vi "Writetofile.vi"(3 "error in (no error)":errorcluster, 4 "Componenet":string, 5 "Write":bool, 6 "Card":i32) -> (0 "error out":errorcluster)   [LabVIEW 2011]
doc: "The vi are saving the current circuit configuration.\n\nThe port White are enable/disable writing to the file, False --> disable writing, True --> enable writing.\n\nThe file are saved on Current VI's Path."
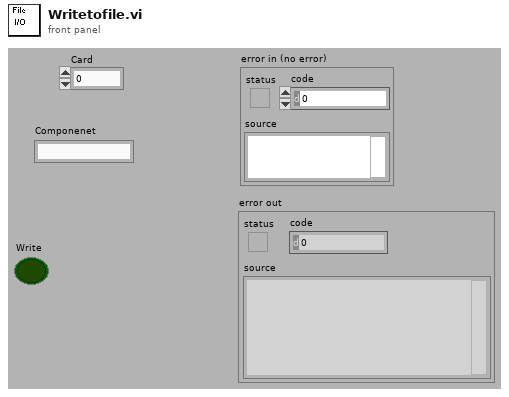
[diagram p1: front panel]
types:
  T1 = cluster{"Card":i32, "Componenet":string, " Format ":string, string[]}
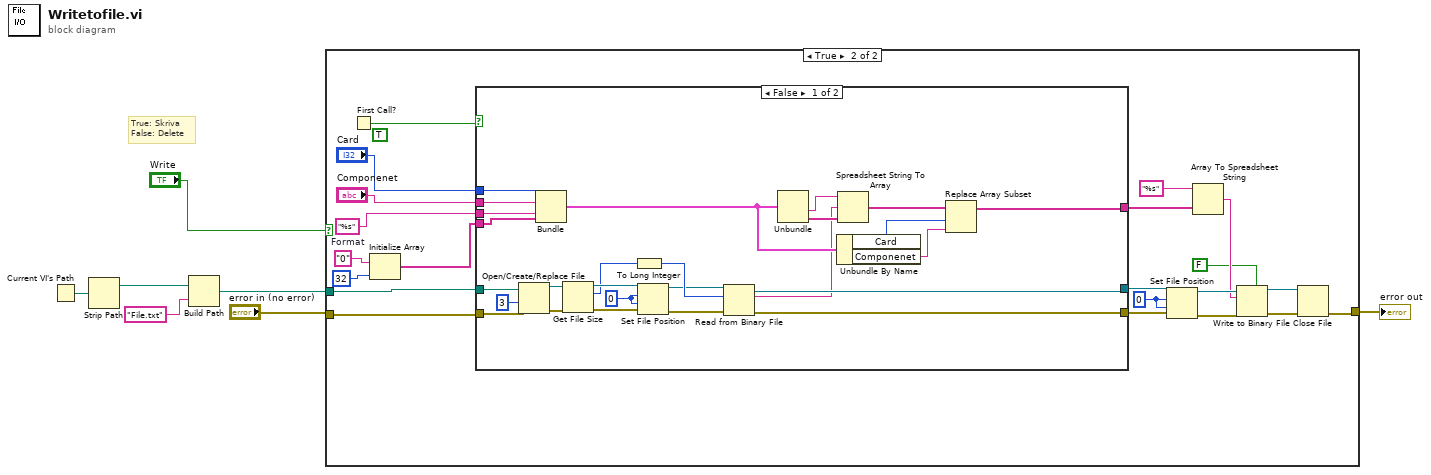
[diagram p0: block diagram]
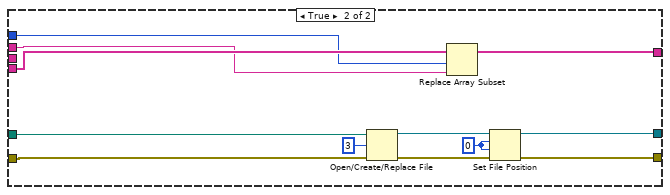
[diagram p3: hidden frame]
diagram:
  # "True: Skriva\nFalse: Delete"
  n1 = Current VI's Path() -> (path=w6:path)
  n2 = Strip Path(path=w6) -> (stripped path=w4:path)  [unwired: 1 out]
  n3 = Build Path(base path=w4, name or relative path="File.txt") -> (appended path=w5:path)
  n4 = case shown="True" "Write" {
    tunnel: [w8 w16] -> w7
    tunnel: w5 -> [_ w15]
    tunnel: "error in (no error)" -> [w8 w14]
    frame False {
    }
    frame True {
      w10 = 0
      w12 = "%s"  # Format
      (unwired) TRUE
      n5 = First Call?() -> (First Call?: T/F=w9:bool)
      n6 = Initialize Array "Initialize Array"("0", 32) -> (w25:string[])
      n7 = case shown="False" w9 {
        tunnel: w14 -> [w31 w67]
        tunnel: "Card" -> [w50 w57]
        tunnel: "Componenet" -> [w49 w56]
        tunnel: w25 -> [w52 w58]
        tunnel: [w54 w66] -> w24
        tunnel: [w34 w62] -> w23
        tunnel: [w32 w61] -> w21
        tunnel: w15 -> [w30 w60]
        tunnel: w12 -> [w53 _]
        frame False {
          w39 = 0
          n8 = Open/Create/Replace File(file path (use dialog)=w30, error in=w31, operation (0:open)=3) -> (refnum out=w44:refnum<file>, error out=w43:errorcluster)  [unwired: 3 in, 1 out]
          n9 = Bundle("Card"=w50, "Componenet"=w49, "Format"=w53, w52) -> (w48:T1)  [unwired: 1 in]
          n10 = Get File Size(file=w44, error in=w43) -> (refnum out=w42:refnum<file>, size (in bytes)=w38:i64, 0:w41:errorcluster)
          n11 = To Long Integer(number=w38) -> (32bit integer=w37:i32)
          n12 = Set File Position(offset (in bytes) (0)=w39, refnum=w42, from (0:start)=w39, error in=w41) -> (refnum out=w36:refnum<file>, error out=w40:errorcluster)
          n13 = Read from Binary File(8:w40, 10:w37, 11:w36) -> (0:w32:errorcluster, 2:w33:string, 3:w34:refnum<file>)  [unwired: 3 in, 1 out]
          n14 = Unbundle(w48) -> ("Format"=w51:string, w45:string[])  [unwired: 2 out]
          n15 = Unbundle By Name(w48) -> ("Card"=w47:i32, "Componenet"=w46:string)
          n16 = Spreadsheet String To Array(format string=w51, spreadsheet string=w33, array type (2D Dbl)=w45) -> (array=w55:string[])  [unwired: 1 in]
          n17 = Replace Array Subset(array=w55, new element=w46, index=w47) -> (w54:string[])
        }
        frame True {
          w63 = 0
          n18 = Open/Create/Replace File(file path (use dialog)=w60, error in=w67, operation (0:open)=3) -> (refnum out=w65:refnum<file>, error out=w64:errorcluster)  [unwired: 3 in, 1 out]
          n19 = Replace Array Subset(array=w58, new element=w56, index=w57) -> (w66:string[])
          n20 = Set File Position(offset (in bytes) (0)=w63, refnum=w65, from (0:start)=w63, error in=w64) -> (refnum out=w62:refnum<file>, error out=w61:errorcluster)
        }
      }
      n21 = Set File Position(offset (in bytes) (0)=w10, refnum=w23, from (0:start)=w10, error in=w21) -> (refnum out=w22:refnum<file>, error out=w20:errorcluster)
      n22 = Array To Spreadsheet String(array=w24, 3:"%s") -> (spreadsheet string=w19:string)  [unwired: 1 in]
      n23 = Write to Binary File(file (use dialog)=w22, data=w19, error in=w20, 5:FALSE) -> (refnum out=w18:refnum<file>, error out=w17:errorcluster)  [unwired: 2 in, 1 out]
      n24 = Close File(refnum=w18, error in=w17) -> (error out=w16:errorcluster)  [unwired: 1 out]
    }
  }
  "error out" <- w7
